vi "Read Raw UTF-8 Path.vi"(9 "UTF-8 Path":refnum<class "UTF-8 Path.lvclass">) -> (1 "Raw UTF-8 Path":T1)   [LabVIEW 2020, in "G-Unicode.lvlib" / "UTF-8 Path.lvclass"]
doc: "Get the UTF-8 encoded path as a LabVIEW path."
uses:
  UTF-8 Path.lvclass
  Raw UTF-8 Path.ctl
  UTF-8 Path.lvclass/UTF-8 Path.ctl
  G-Unicode.lvlib
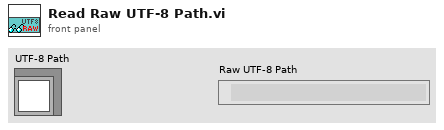
[diagram p1: front panel]
types:
  T1 = typedef "G-Unicode.lvlib/Raw UTF-8 Path.ctl" = path
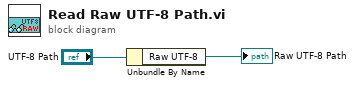
[diagram p0: block diagram]
diagram:
  n1 = Unbundle By Name("UTF-8 Path") -> ("Raw UTF-8"=→"Raw UTF-8 Path":T1)
